vi "Read Laser Status.vi"(10 "error in":errorcluster, 11 "reference in":refnum<k7>) -> (0 "Laser Current":sgl, 1 "Safety interlock":bool, 2 "Key Switch enabled":bool, 3 "output enabled":bool, 4 "error out":errorcluster, 5 "reference out":refnum<k7>)   [LabVIEW 2014]
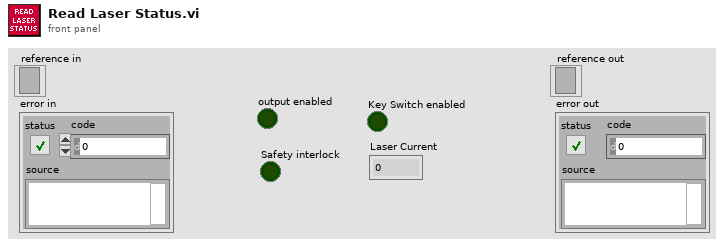
[diagram p1: front panel]
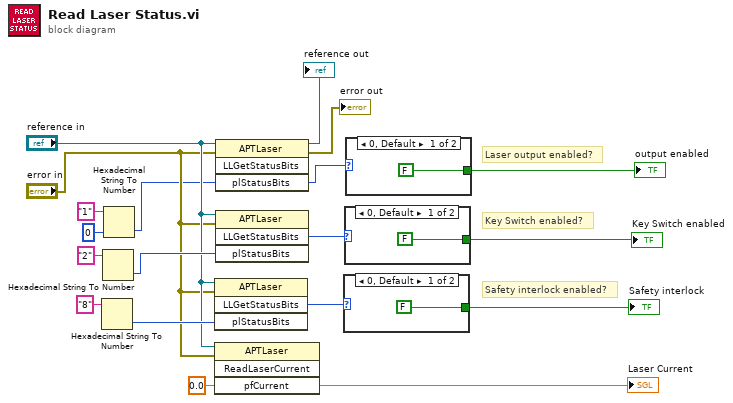
[diagram p0: block diagram]
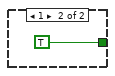
[diagram p2: hidden frame]
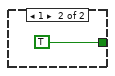
[diagram p3: hidden frame]
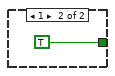
[diagram p4: hidden frame]
diagram:
  # "Safety interlock enabled?"
  # "Key Switch enabled?"
  # "Laser output enabled?"
  n1 = Hexadecimal String To Number(string="8") -> (number=w15:u32)  [unwired: 2 in, 1 out]
  n2 = Hexadecimal String To Number(string="2") -> (number=w17:u32)  [unwired: 2 in, 1 out]
  n3 = Hexadecimal String To Number(string="1", default (0uL)=u32 0 ("default (0 U32)")) -> (number=w2:u32)  [unwired: 1 in, 1 out]
  n4 = invoke class="APTLaser" method="LLGetStatusBits"(reference="reference in", error in="error in", "plStatusBits"=w15) -> ("LLGetStatusBits"=w4:i32)  [unwired: 1 in, 3 out]
  n5 = invoke class="APTLaser" method="ReadLaserCurrent"(reference="reference in", error in="error in", "pfCurrent"=sgl 0.0) -> ("pfCurrent"=→"Laser Current":sgl)  [unwired: 1 in, 3 out]
  n6 = invoke class="APTLaser" method="LLGetStatusBits"(reference="reference in", error in="error in", "plStatusBits"=w2) -> (reference out=→"reference out":refnum<k7>, error out=→"error out":errorcluster, "plStatusBits"=w1:i32)  [unwired: 1 in, 1 out]
  n7 = invoke class="APTLaser" method="LLGetStatusBits"(reference="reference in", error in="error in", "plStatusBits"=w17) -> ("LLGetStatusBits"=w5:i32)  [unwired: 1 in, 3 out]
  n8 = case shown="0, Default" w4 {
    tunnel: [FALSE TRUE] -> w12
    frame 0, Default {
    }
    frame 1 {
    }
  }
  "Safety interlock" <- w12
  n9 = case shown="0, Default" w5 {
    tunnel: [FALSE TRUE] -> w13
    frame 0, Default {
    }
    frame 1 {
    }
  }
  "Key Switch enabled" <- w13
  n10 = case shown="0, Default" w1 {
    tunnel: [FALSE TRUE] -> w14
    frame 0, Default {
    }
    frame 1 {
    }
  }
  "output enabled" <- w14
